vi "DMM_DC-RMS Voltage Meas Format Function Range.vi"(0 "DMM Handle In":refnum<k15>, 5 "Function Settings In":T4={"Range and Function"=enum."DC Voltage Auto Range", "Resolution in Digits"=5.5} {"Resolution in Digits" items=["3 1/2"=3.5, "4 1/2"=4.5, "5 1/2"=5.5, "6 1/2"=6.5, "7 1/2"=7.5]}, 11 "error in":errorcluster) -> (4 "DMM Handle Out":refnum<k15>, 6 "Function Settings Out":T3={"Range"=0.0, "Function"=enum."DC Volts", "Freq_Period AC Range"=0.0, "Resolution in Digits"=5.5} {"Resolution in Digits" items=["3 1/2"=3.5, "4 1/2"=4.5, "5 1/2"=5.5, "6 1/2"=6.5, "7 1/2"=7.5]}, 15 "error out":errorcluster)   [LabVIEW 2021, in "DMM_DC-RMS Voltage Measurement.lvlib"]
doc: "Utilizes the function settings input to select the particular function and range used for the measurement and format the output string displayed in the measurement output cluster."
uses:
  DMM_DC-RMS Voltage Measurement.lvlib
  Typedefs/Function Settings.ctl
  <instrlib>/niDMM/nidmm.llb/niDMM Resolution in Digits.ctl
  <instrlib>/niDMM/nidmm.llb/niDMM Function.ctl
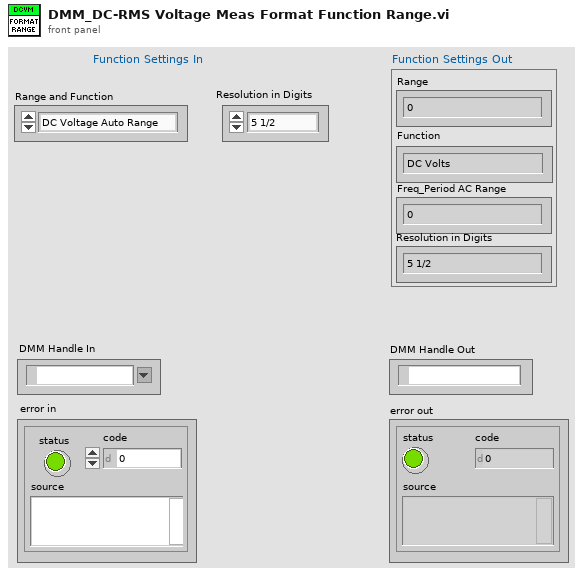
[diagram p1: front panel]
types:
  T1 = typedef "niDMM Function.ctl" = enum16{"DC Volts", "AC Volts", "DC Current", "AC Current", "2-wire Resistance", "4-wire Resistance", "Diode", "Frequency", "Period", "AC Volts DC Coupled", "Capacitance", "Inductance", "Temperature"}
  T2 = typedef "niDMM Resolution in Digits.ctl" = dbl
  T3 = cluster{"Range":dbl, "Function":T1, "Freq_Period AC Range":dbl, "Resolution in Digits":T2}
  T4 = typedef "DMM_DC-RMS Voltage Measurement.lvlib/Function Settings.ctl" = cluster{"Range and Function":enum16{"DC Voltage Auto Range", "DC 100 mV", "DC 1 V ", "DC 10 V", "DC 100 V", "DC 300 V", " ", "AC Voltage Auto Range", "AC 50 mV", "AC 200 mV", "AC 500 mV", "AC 2 V", "AC 5 V", "AC 20 V", "AC 50 V", "AC 300 V"}, "Resolution in Digits":T2}
  T5 = enum16{"DC Voltage Auto Range", "DC 100 mV", "DC 1 V ", "DC 10 V", "DC 100 V", "DC 300 V", " ", "AC Voltage Auto Range", "AC 50 mV", "AC 200 mV", "AC 500 mV", "AC 2 V", "AC 5 V", "AC 20 V", "AC 50 V", "AC 300 V"}
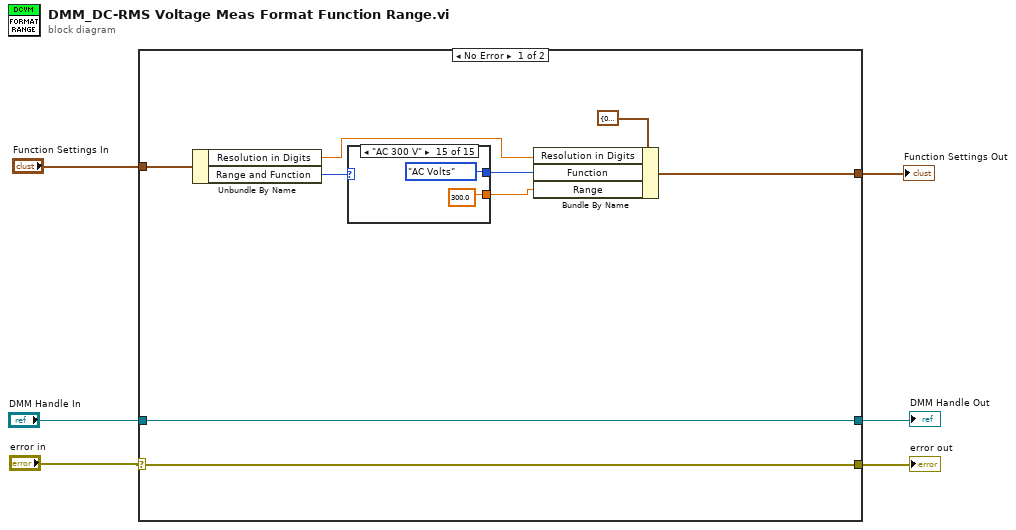
[diagram p0: block diagram]
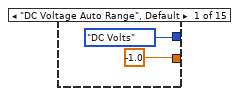
[diagram p2: hidden frame]
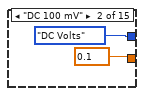
[diagram p3: hidden frame]
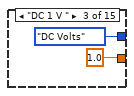
[diagram p4: hidden frame]
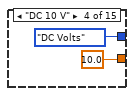
[diagram p5: hidden frame]
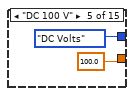
[diagram p6: hidden frame]
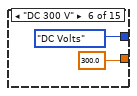
[diagram p7: hidden frame]
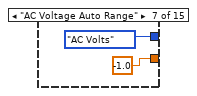
[diagram p8: hidden frame]
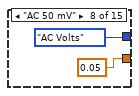
[diagram p9: hidden frame]
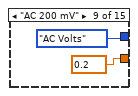
[diagram p10: hidden frame]
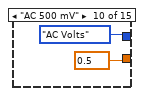
[diagram p11: hidden frame]
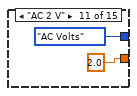
[diagram p12: hidden frame]
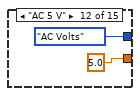
[diagram p13: hidden frame]
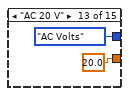
[diagram p14: hidden frame]
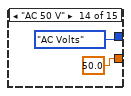
[diagram p15: hidden frame]
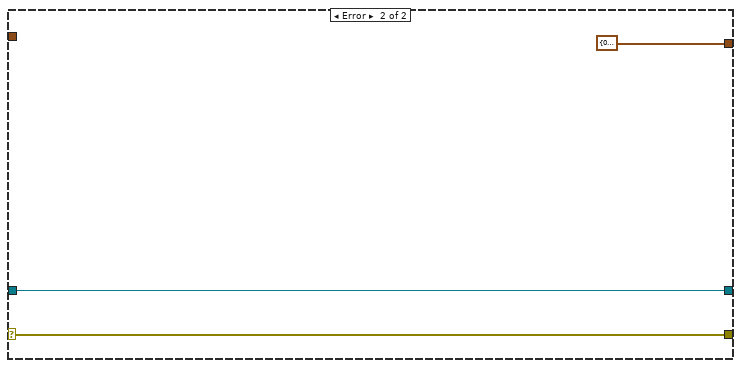
[diagram p16: hidden frame]
diagram:
  n1 = case shown="No Error" "error in" {
    selector: "error in" -> [w13 w47]
    tunnel: "Function Settings In" -> [w15 _]
    tunnel: [w9 T3 {"Range"=0.1, "Function"=enum."DC Volts", "Freq_Period AC Range"=0.1, "Resolution in Digits"=5.5} ("Function Settings")] -> w1
    tunnel: [w13 w47] -> w5
    tunnel: [w12 w48] -> w3
    tunnel: "DMM Handle In" -> [w12 w48]
    frame No Error {
      n2 = Unbundle By Name(w15) -> ("Resolution in Digits"=w14:T2, "Range and Function"=w11:T5)
      n3 = case shown="\"AC 300 V\"" w11 {
        tunnel: [niDMM_Function."DC Volts" ("Function") niDMM_Function."DC Volts" ("Function") niDMM_Function."DC Volts" ("Function") niDMM_Function."DC Volts" ("Function") niDMM_Function."DC Volts" ("Function") niDMM_Function."DC Volts" ("Function") niDMM_Function."AC Volts" ("Function") niDMM_Function."AC Volts" ("Function") niDMM_Function."AC Volts" ("Function") niDMM_Function."AC Volts" ("Function") niDMM_Function."AC Volts" ("Function") niDMM_Function."AC Volts" ("Function") niDMM_Function."AC Volts" ("Function") niDMM_Function."AC Volts" ("Function") niDMM_Function."AC Volts" ("Function")] -> w10
        tunnel: [-1.0 ("Range") 0.1 ("Range") 1.0 ("Range") 10.0 ("Range") 100.0 ("Range") 300.0 ("Range") -1.0 ("Range") 0.05 ("Range") 0.2 ("Range") 0.5 ("Range") 2.0 ("Range") 5.0 ("Range") 20.0 ("Range") 50.0 ("Range") 300.0 ("Range")] -> w7
        frame "DC Voltage Auto Range", Default {
        }
        frame "DC 100 mV" {
        }
        frame "DC 1 V " {
        }
        frame "DC 10 V" {
        }
        frame "DC 100 V" {
        }
        frame "DC 300 V" {
        }
        frame "AC Voltage Auto Range" {
        }
        frame "AC 50 mV" {
        }
        frame "AC 200 mV" {
        }
        frame "AC 500 mV" {
        }
        frame "AC 2 V" {
        }
        frame "AC 5 V" {
        }
        frame "AC 20 V" {
        }
        frame "AC 50 V" {
        }
        frame "AC 300 V" {
        }
      }
      n4 = Bundle By Name(cluster=T3 {"Range"=0.1, "Function"=enum."DC Volts", "Freq_Period AC Range"=0.1, "Resolution in Digits"=5.5} ("Function Settings"), "Resolution in Digits"=w14, "Function"=w10, "Range"=w7) -> (w9:T3)
    }
    frame Error {
    }
  }
  "error out" <- w5
  "DMM Handle Out" <- w3
  "Function Settings Out" <- w1
